vi "string.vi"() -> ()   [LabVIEW 2015]
panel:
  out "appended array real time":string[](array[string])
  out "Array wrong timing":string[](array[string])
  out "Numeric Control":i32
  out "after substring":string
  out "before substring":string
  out "number of replacements":i32
  in  "regular expression":string="_"
  in  "String input":string="xfiles_season1_episode1_@silu_DTS_1040p.mkv"
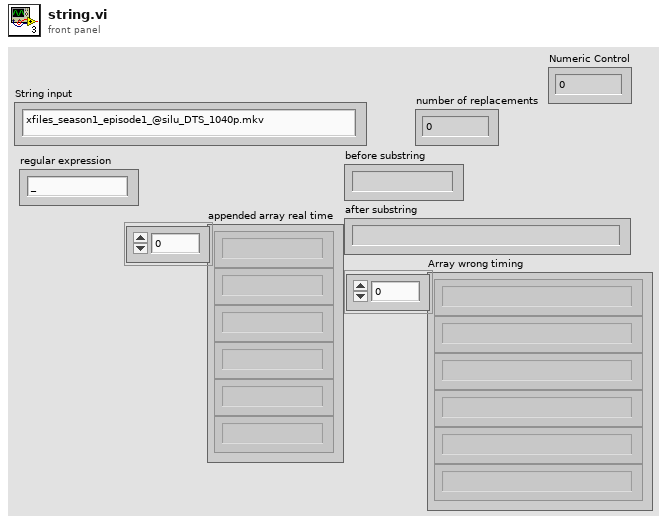
[diagram p1: front panel]
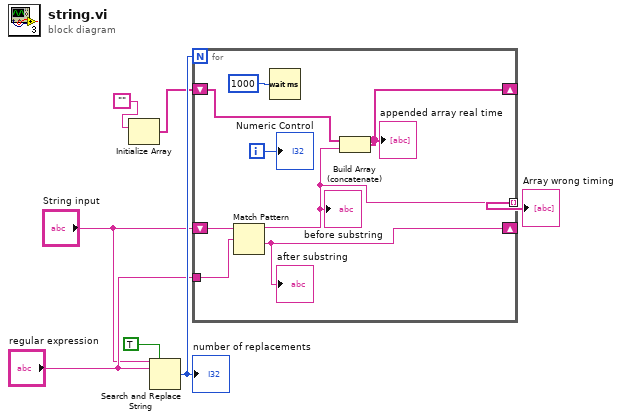
[diagram p0: block diagram]
diagram:
  n1 = Initialize Array("") -> (w1:string[])  [unwired: 1 in]
  n2 = Search and Replace String(replace all?=TRUE ("replace all? (F)"), input string="String input", search string="regular expression") -> (number of replacements=w6:i32)  [unwired: 5 in, 3 out]
  "number of replacements" <- w6
  n3 = for {
    N: w6 -> [_]
    tunnel: "regular expression" -> [w15]
    shift-right: [w12] -> _
    shift-left: "String input" -> [w13]
    tunnel: [w8] -> w3 mode=indexing
    shift-right: [w10] -> _
    shift-left: w1 -> [w9]
    i -> [w11]
    n4 = Match Pattern(string=w13, regular expression=w15) -> (before substring=w8:string, after substring=w12:string)  [unwired: 1 in, 2 out]
    "before substring" <- w8
    "after substring" <- w12
    n5 = Wait (ms)(milliseconds to wait=u32 1000) -> ()  [unwired: 1 out]
    n6 = Build Array (concatenate)(w9, w8) -> (w10:string[])
    "appended array real time" <- w10
    "Numeric Control" <- w11
  }
  "Array wrong timing" <- w3
